vi "Disconnect.vi"(8 "error in (no error)":errorcluster, 11 "reference in":refnum<class "Camera_IMAQdx.lvclass">) -> (0 "error out":errorcluster, 3 "reference out":refnum<class "Camera_IMAQdx.lvclass">)   [LabVIEW 2017, in "Camera_IMAQdx.lvclass"]
doc: "Closes connection to an IMAQ camera"
uses:
  Camera_IMAQdx.lvclass
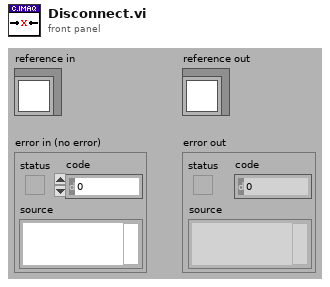
[diagram p1: front panel]
types:
  T1 = typedef "IMAQdx.ctl" = refnum<k21>
  T2 = typedef "IMAQ Image.ctl" = refnum<image>
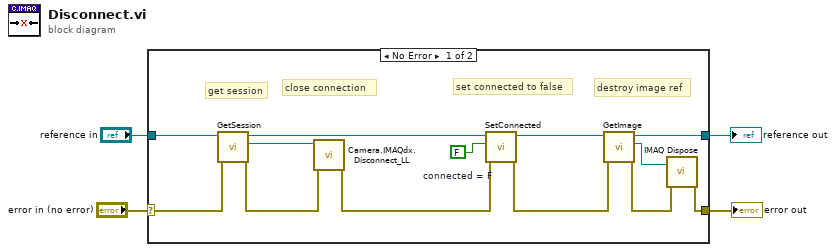
[diagram p0: block diagram]
diagram:
  n1 = case shown="No Error" "error in (no error)" {
    selector: "error in (no error)" -> [w17 w19]
    tunnel: [w5 w19] -> w3
    tunnel: [w9 w18] -> w1
    tunnel: "reference in" -> [w15 w18]
    frame No Error {
      w11 = FALSE  # connected = F
      # "destroy image ref"
      # "set connected to false"
      # "close connection"
      # "get session"
      n2 = call "GetSession.vi"("error in (no error)"=w17, "reference in"=w15) -> ("error out"=w16:errorcluster, "Session"=w13:T1, "reference out"=w14:refnum<class "Camera_IMAQdx.lvclass">)  [unwired: 7 in]
      n3 = call "Camera.IMAQdx.Disconnect_LL.vi"("Error In"=w16, "Session In"=w13) -> ("Error Out"=w10:errorcluster)  [unwired: 9 in]
      n4 = call "SetConnected.vi"("error in (no error)"=w10, "Connected"=w11, "reference in"=w14) -> ("error out"=w7:errorcluster, "reference out"=w12:refnum<class "Camera_IMAQdx.lvclass">)  [unwired: 7 in]
      n5 = call "GetImage.vi"("error in (no error)"=w7, "reference in"=w12) -> ("error out"=w6:errorcluster, "Image"=w8:T2, "reference out"=w9:refnum<class "Camera_IMAQdx.lvclass">)  [unwired: 7 in]
      n6 = call "IMAQ Dispose"("Image"=w8, "error in (no error)"=w6) -> ("error out"=w5:errorcluster)  [unwired: 4 in]
    }
    frame Error {
    }
  }
  "error out" <- w3
  "reference out" <- w1
